vi "Compare with Current time.vi"(9 "Note Events":T1[](array[typedef]), 10 "Numeric Control 2":i32, 11 "Numeric Control":u32) -> (2 "Array":T1, 3 "Boolean":bool)   [LabVIEW 2016]
uses:
  Notes.ctl
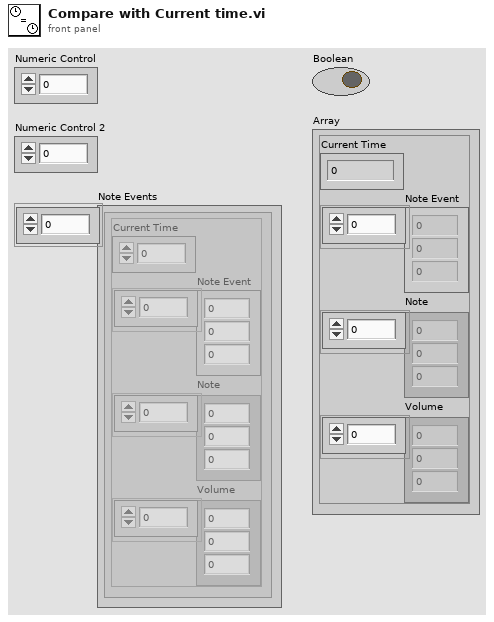
[diagram p1: front panel]
types:
  T1 = typedef "Notes.ctl" = cluster{"Current Time":u32, "Note Event":u32[], "Note":u32[], "Volume":u32[]}
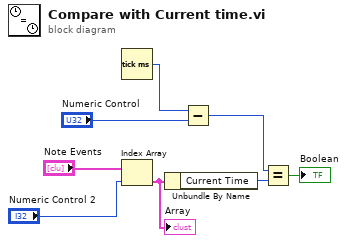
[diagram p0: block diagram]
diagram:
  n1 = Tick Count (ms)() -> (millisecond timer value=w2:u32)
  n2 = Index Array(array="Note Events", index="Numeric Control 2") -> (element=w4:T1)
  "Array" <- w4
  n3 = Unbundle By Name(w4) -> ("Current Time"=w1:u32)
  n4 = Subtract(x=w2, y="Numeric Control") -> (x-y=w3:u32)
  n5 = Equal?(x=w3, y=w1) -> (x = y?=→"Boolean":bool)
